vi "Auto Rotate to Angle Gyro.vi"(2 "Drive to Angle":dbl format="%.2f") -> (0 "Rotational Adjustment":dbl format="%.2f")   [LabVIEW 2020]
uses:
  Robot Global Data.vi
  <vilib>/addons/control/pid/pid.llb/PID (DBL).vi
  <vilib>/addons/control/pid/NI_PID_pid.lvlib
panel:
  out "NavX Comp Yaw":dbl
  in  "PID gains":T1={"proportional gain (Kc)"=0.005, "integral time (Ti, min)"=0.0, "derivative time (Td, min)"=0.0}
  in  "output range":cluster{"output high":dbl, "output low":dbl}={"output high"=0.15, "output low"=-0.15} {"output low" format="%.2f"; "output high" format="%.2f"}
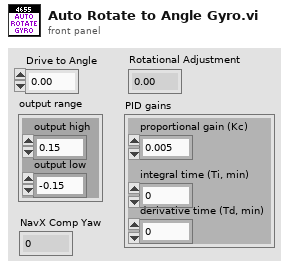
[diagram p1: front panel]
types:
  T1 = cluster{"proportional gain (Kc)":dbl, "integral time (Ti, min)":dbl, "derivative time (Td, min)":dbl}
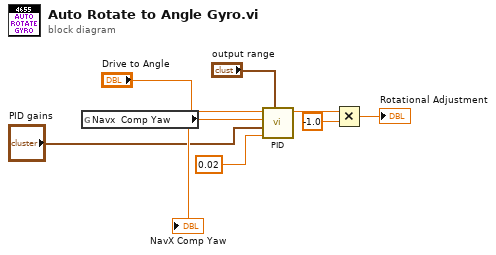
[diagram p0: block diagram]
diagram:
  n1 = global read "Robot Global Data.vi" "Navx  Comp Yaw"() -> (w7:dbl)
  "NavX Comp Yaw" <- w7
  n2 = call-poly <vilib>:"PID.vi"("output range"="output range", "dt (s)"=0.02, "PID gains"="PID gains", "process variable"=w7, "setpoint"="Drive to Angle") -> ("output"=w2:dbl)  [unwired: 5 in, 1 out]
  n3 = Multiply(x=w2, y=-1.0) -> (x*y=→"Rotational Adjustment":dbl)
